vi "Configure Bus Source (LIN).vi"(0 "VISA resource name":refnum<visa-resource-name>, 1 "LIN Polarity (0: Normal)":u16(ring) items=["Normal", "Invert"], 2 "LIN Standard (0: V1X)":u16(ring) items=["V1X", "V2X", "Mixed"], 5 "BUS Number (9: Bus 1)":u16(ring)=9 items=["Bus 1"=9, "Bus 2"=10, "Bus 3"=11, "Bus 4"=12], 7 "LIN Source (0: Channel 1)":u16(ring) items=["Channel 1", "Channel 2", "Channel 3", "Channel 4"], 9 "Bit Rate (9600)":i32=9600, 11 "error in (no error)":errorcluster, 12 "LIN ID Format (0: V1X)":u16(ring) items=["No Parity", "Parity"], 13 "LIN Sample Point (50)":i32=50) -> (4 "VISA resource name out":refnum<visa-resource-name>, 15 "error out":errorcluster)   [LabVIEW 2010, in "Tektronix DPO MSO 2000 4000 Series.lvlib"]
doc: "This VI configures the LIN bus.\n\n<B>Note:</B> This VI is only valid if you have installed the DPO3AUTO application module."
uses:
  <instrlib>/Tektronix DPO MSO 2000 4000 Series/Tektronix DPO MSO 2000 4000 Series.lvlib
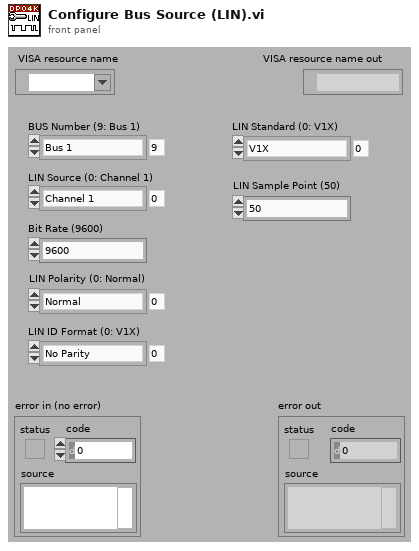
[diagram p1: front panel]
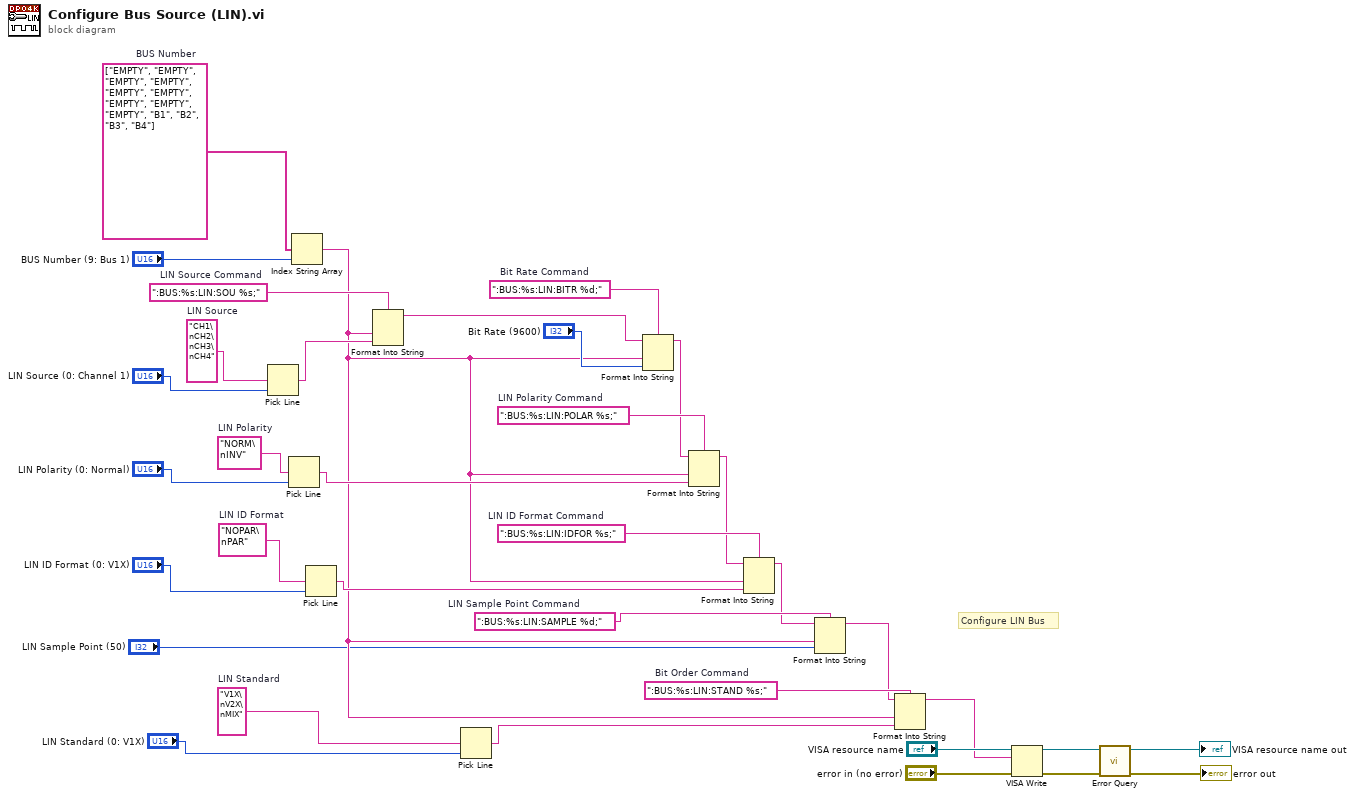
[diagram p0: block diagram]
diagram:
  w4 = ":BUS:%s:LIN:SAMPLE %d;"  # LIN Sample Point Command
  w9 = "NOPAR\nPAR"  # LIN ID Format
  w12 = "NORM\nINV"  # LIN Polarity
  w15 = "CH1\nCH2\nCH3\nCH4"  # LIN Source
  w17 = ":BUS:%s:LIN:IDFOR %s;"  # LIN ID Format Command
  w19 = ":BUS:%s:LIN:POLAR %s;"  # LIN Polarity Command
  w21 = ":BUS:%s:LIN:BITR %d;"  # Bit Rate Command
  w31 = "V1X\nV2X\nMIX"  # LIN Standard
  w30 = ":BUS:%s:LIN:STAND %s;"  # Bit Order Command
  w33 = ":BUS:%s:LIN:SOU %s;"  # LIN Source Command
  w34 = string[] ["EMPTY", "EMPTY", "EMPTY", "EMPTY", "EMPTY", "EMPTY", "EMPTY", "EMPTY", "EMPTY", "B1", "B2", "B3", "B4"]  # BUS Number
  # "Configure LIN Bus"
  n1 = Pick Line(multi-line string=w15, line index="LIN Source (0: Channel 1)") -> (output string=w13:string)  [unwired: 1 in]
  n2 = Pick Line(multi-line string=w12, line index="LIN Polarity (0: Normal)") -> (output string=w10:string)  [unwired: 1 in]
  n3 = Index String Array(1:"BUS Number (9: Bus 1)", 2:w34) -> (0:w5:string)  [unwired: 1 in]
  n4 = Pick Line(multi-line string=w9, line index="LIN ID Format (0: V1X)") -> (output string=w7:string)  [unwired: 1 in]
  n5 = Format Into String(format string=w33, w5, w13) -> (resulting string=w32:string)  [unwired: 2 in, 1 out]
  n6 = Pick Line(multi-line string=w31, line index="LIN Standard (0: V1X)") -> (output string=w22:string)  [unwired: 1 in]
  n7 = Format Into String(format string=w21, initial string=w32, w5, "Bit Rate (9600)") -> (resulting string=w18:string)  [unwired: 1 in, 1 out]
  n8 = Format Into String(format string=w19, initial string=w18, w5, w10) -> (resulting string=w16:string)  [unwired: 1 in, 1 out]
  n9 = Format Into String(format string=w17, initial string=w16, w5, w7) -> (resulting string=w2:string)  [unwired: 1 in, 1 out]
  n10 = Format Into String(format string=w4, initial string=w2, w5, "LIN Sample Point (50)") -> (resulting string=w1:string)  [unwired: 1 in, 1 out]
  n11 = Format Into String(format string=w30, initial string=w1, w5, w22) -> (resulting string=w27:string)  [unwired: 1 in, 1 out]
  n12 = VISA Write(VISA resource name="VISA resource name", write buffer=w27, error in (no error)="error in (no error)") -> (VISA resource name out=w26:refnum<visa-resource-name>, error out=w25:errorcluster)  [unwired: 1 out]
  n13 = call <instrlib>:"Error Query.vi"("error in (no error)"=w25, "VISA resource name"=w26) -> ("error out"=→"error out":errorcluster, "VISA resource name out"=→"VISA resource name out":refnum<visa-resource-name>)  [unwired: 6 in, 2 out]
